vi "Index Array.vi"(8 "错误输入":errorcluster, 9 "Inices(>=1D)":u32[](array[numeric]), 10 "Index(1D)":u32, 11 "MultiD Array":variant) -> (0 "错误输出":errorcluster, 2 "Array Element":variant)   [LabVIEW 2012, in "TD Tools.lvlib"]
uses:
  TD Tools.lvlib
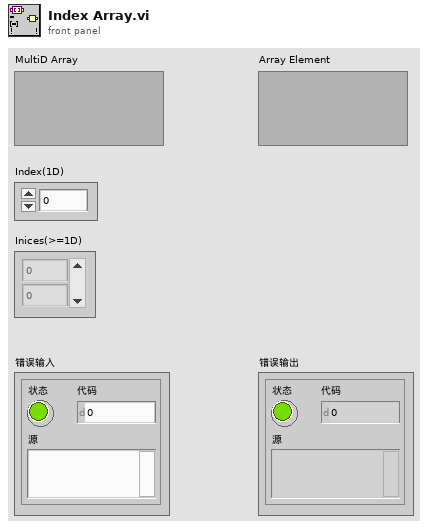
[diagram p1: front panel]
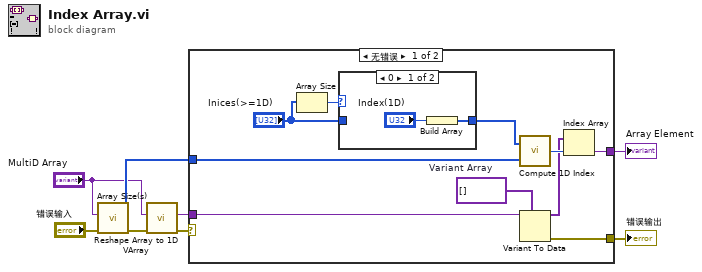
[diagram p0: block diagram]
diagram:
  n1 = call "Array Size(s).vi"("错误输入"="错误输入", "Array"="MultiD Array") -> ("错误输出"=w7:errorcluster, "Size(s)"=w8:u32[])  [unwired: 7 in, 1 out]
  n2 = call "Reshape Array to 1D VArray.vi"("error in (no error)"=w7, "MultiD Array"="MultiD Array") -> ("error out"=w5:errorcluster, "1D VArray"=w6:variant)  [unwired: 7 in, 1 out]
  n3 = case shown="无错误" w5 {
    selector: w5 -> [_ w22]
    tunnel: [w10 w22] -> w3
    tunnel: w6 -> [w18 _]
    tunnel: w8 -> [w15 _]
    tunnel: [w11 _] -> w2
    frame No Error {
      w17 = variant[] []  # Variant Array
      n4 = Array Size(array="Inices(>=1D)") -> (size(s)=w16:i32)
      n5 = case shown="0" w16 {
        tunnel: [w20 w21] -> w14
        tunnel: "Inices(>=1D)" -> [_ w21]
        frame 0 {
          n6 = Build Array("Index(1D)") -> (w20:u32[])
        }
        frame Default {
        }
      }
      n7 = call "Compute 1D Index.vi"("Size(s)"=w15, "Indices"=w14) -> ("1D Index"=w13:i32)
      n8 = Variant To Data(type=w17, Variant=w18) -> (data=w12:variant[], error out=w10:errorcluster)  [unwired: 1 in]
      n9 = Index Array(array=w12, index=w13) -> (element=w11:variant)
    }
    frame Error {
    }
  }
  "Array Element" <- w2
  "错误输出" <- w3
